vi "simulation.vi"() -> ()   [LabVIEW 2014]
uses:
  <vilib>/userdefined/High Color/IMAQdx.ctl
  <vilib>/vision/driver/IMAQdx.llb/IMAQdx Camera Control Mode.ctl
  <vilib>/vision/driver/NI_Vision_Acquisition_Software.lvlib
  <resource>/objmgr/imaqdx.rc
panel:
  out "length":i32
  out "Image 2":T1(plugin-control)
  in  "Quality (750)":i32=750
  in  "Type of Flatten (Image and Vision Info)":i32(ring)=1 items=["Image", "Image and Vision Info", "Reference to Image"]
  in  "Compression (None)":i32(ring) items=["None", "JPEG", "PACKED BINARY"]
  out "error out":errorcluster
  out "Image":T1(plugin-control)
  in  "millisecond multiple":u32
  in  "Camera Control Mode":T2
  in  "Session In":T3
  in  "VideoMode":u32
  in  "stop":bool
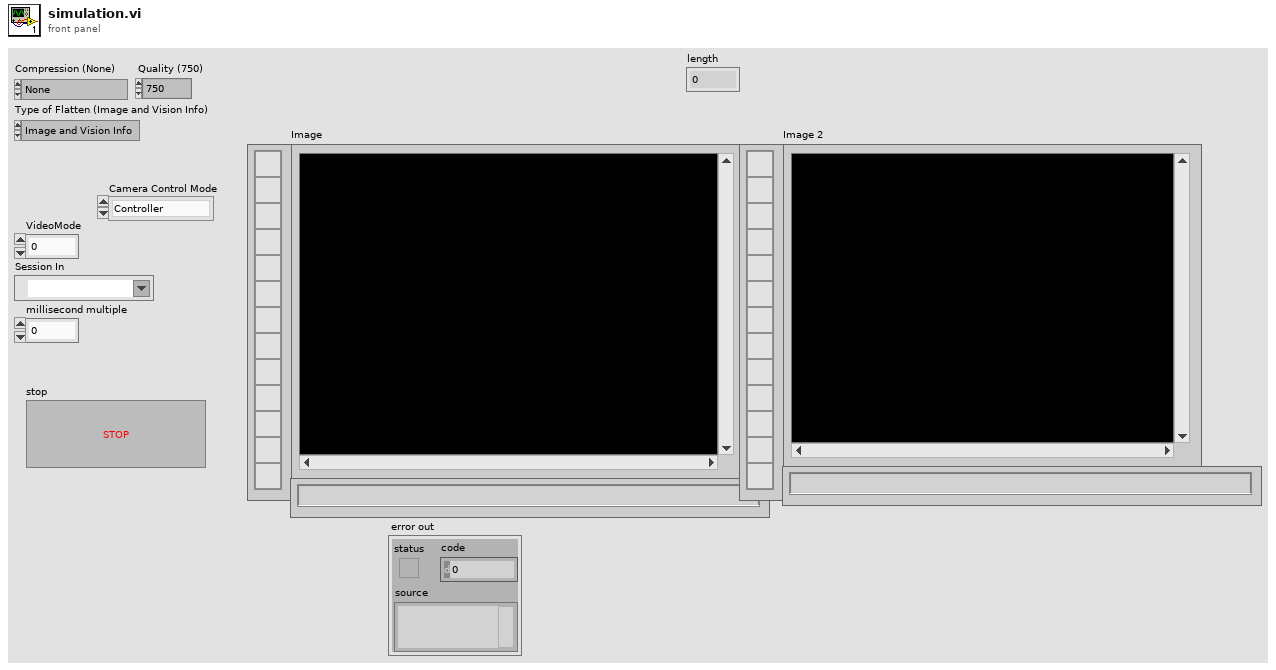
[diagram p1: front panel]
types:
  T1 = typedef "IMAQ Image.ctl" = refnum<image>
  T2 = typedef "NI_Vision_Acquisition_Software.lvlib/IMAQdx Camera Control Mode.ctl" = enum32{"Controller", "Listener"}
  T3 = typedef "IMAQdx.ctl" = refnum<k21>
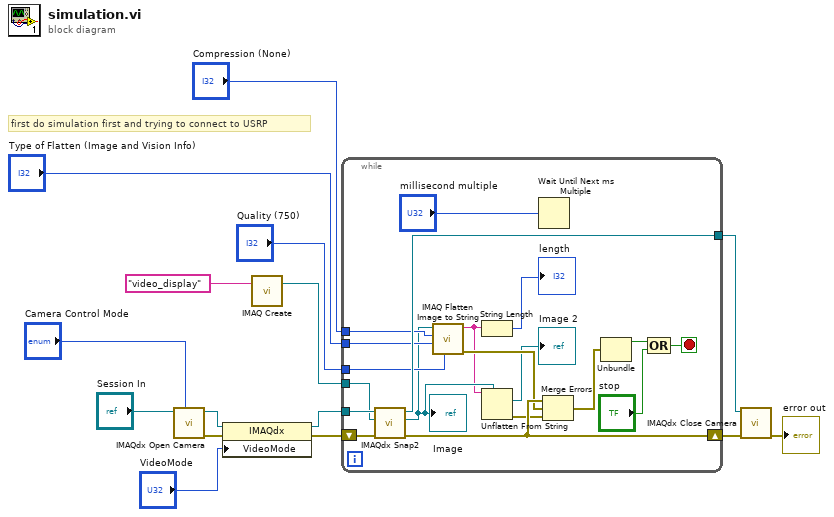
[diagram p0: block diagram]
diagram:
  # "first do simulation first and trying to connect to USRP"
  n1 = call <vilib>:"IMAQdx Open Camera.vi"("Camera Control Mode"="Camera Control Mode", "Session In"="Session In") -> ("error out"=w14:errorcluster, "Session Out"=w15:T3)  [unwired: 8 in]
  n2 = property class="IMAQdx"(reference=w15, error in=w14, "VideoMode"="VideoMode") -> (reference out=w10:T3, error out=w9:errorcluster)
  n3 = call "IMAQ Create"("Image Name"="video_display") -> ("New Image"=w7:T1)  [unwired: 4 in, 1 out]
  n4 = while {
    tunnel: w10 -> [w33]
    shift-right: [w27] -> w5
    shift-left: w9 -> [w32]
    tunnel: w7 -> [w31]
    tunnel: [w30] -> w6
    tunnel: "Compression (None)" -> [w29]
    tunnel: "Type of Flatten (Image and Vision Info)" -> [w28]
    tunnel: "Quality (750)" -> [w21]
    stop <- w22 stop-if-true
    n5 = call <vilib>:"IMAQdx Snap2.vi"("error in"=w32, "Image In"=w31, "Session In"=w33) -> ("error out"=w27:errorcluster, "Image Out"=w20:T1, "Session Out"=w30:T3)  [unwired: 6 in]
    "Image" <- w20
    n6 = call "IMAQ Flatten Image to String"("Quality (750)"=w21, "Type of Flatten (Image and Vision Info)"=w28, "Compression (None)"=w29, "Image"=w20) -> ("error out"=w26:errorcluster, "Data String"=w17:string)  [unwired: 6 in]
    n7 = String Length(string=w17) -> (length=→"length":i32)
    n8 = Unflatten From String(type=w20, binary string=w17) -> (value=→"Image 2":T1, error out=w18:errorcluster)  [unwired: 3 in, 1 out]
    n9 = Wait Until Next ms Multiple(millisecond multiple="millisecond multiple") -> ()  [unwired: 1 out]
    n10 = Merge Errors(w27, w26, w18) -> (w25:errorcluster)
    n11 = Unbundle(w25) -> ("status"=w23:bool)  [unwired: 2 out]
    n12 = Compound Arithmetic op=OR(w23, "stop") -> (w22:bool)
  }
  n13 = call <vilib>:"IMAQdx Close Camera.vi"("error in"=w5, "Session In"=w6) -> ("error out"=→"error out":errorcluster)  [unwired: 9 in]
